vi "挥发酚插入数据.vi"(1 "data":T3 {"单位" items=["ug/L", "mg/L", "ppm", "mg/m3", "cm", "ppb", "ug/m3", "%", "nmol/mol", "umol/mol", "MPN/L", "MPN/100ml", "ng/m3", "NTU", "无量纲", "ms/cm", "us/cm"]}, 2 "挥发酚关键参数":T2, 3 "SN":string, 5 "table":string, 7 "测量模式":T4(ring)=enum."水样测试", 9 "数据类型":string(combo)="N", 11 "error in (no error)":errorcluster) -> (15 "error out":errorcluster)   [LabVIEW 2016, in "挥发酚.lvlib"]
uses:
  <vilib>/Utility/error.llb/DialogType.ctl
panel:
  in  "data2":T1={"时间"=timestamp(0 s since 1904-01-01), "测量模式"="水样测试", "数据类型"="N", "检测值"=0.0, "单位"="mg/L", "数据标识"="N", "X0"=0.0, "标样参考值"=0.0, "跨度值"=0.0, "因子编码"="", "X^2"=0.0, "X"=0.0, "B 2"=0.0, "测量量程"=0.0, "测量检出限"=0.0, "测量精度"=0.0, "测量间隔"=0.0, "消解温度"=0.0, "消解时长"=0.0, "三项式系数"=0.0, "二次多项式系数"=0.0, "曲线斜率"=0.0, "曲线截距"=0.0, "线性相关系数"=0.0, "空白校准时间"=timestamp(0 s since 1904-01-01), "标样校准时间"=timestamp(0 s since 1904-01-01), "测量信号值"=0.0, "稀释倍数"=0.0, "量程系数"=0.0, "LastTime"=timestamp(0 s since 1904-01-01), "量程标识"=""}
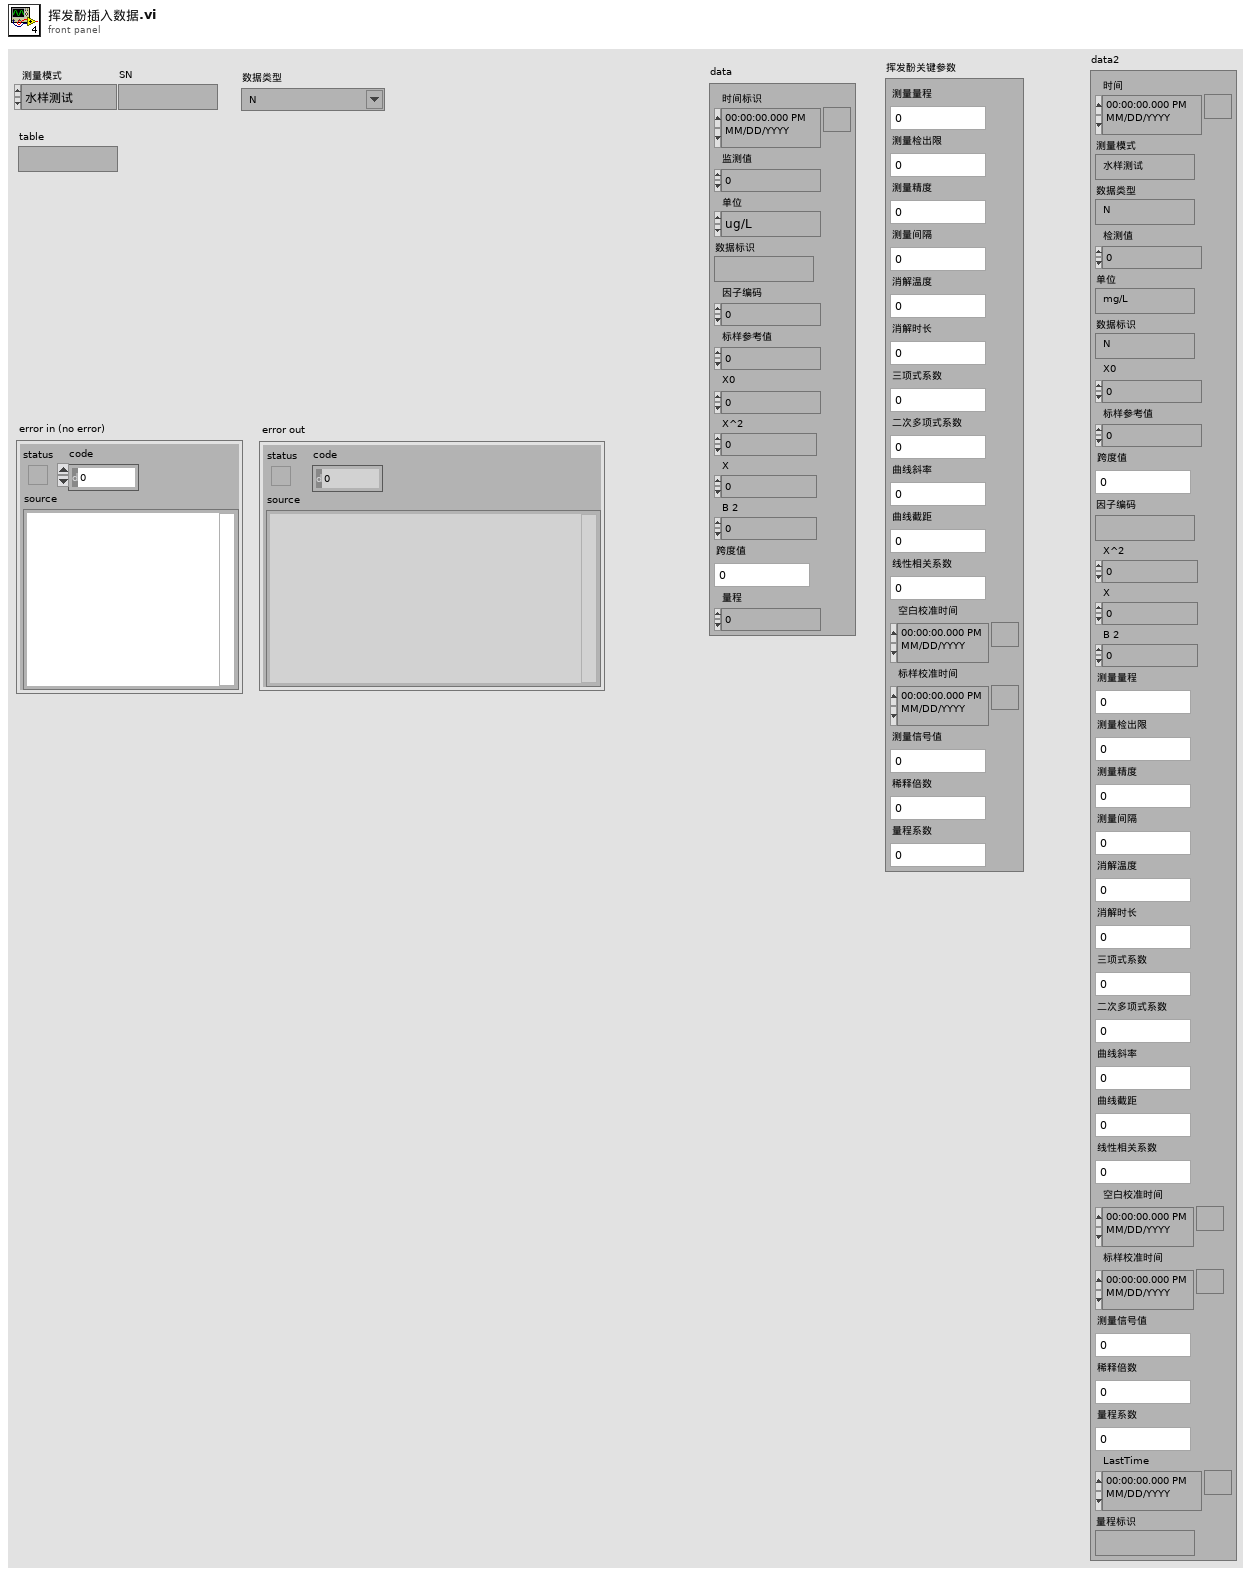
[diagram p1: front panel]
types:
  T1 = cluster{"时间":timestamp, "测量模式":string, "数据类型":string, "检测值":sgl, "单位":string, "数据标识":string, "X0":sgl, "标样参考值":sgl, "跨度值":sgl, "因子编码":string, "X^2":sgl, "X":sgl, "B 2":sgl, "测量量程":sgl, "测量检出限":sgl, "测量精度":sgl, "测量间隔":sgl, "消解温度":sgl, "消解时长":sgl, "三项式系数":sgl, "二次多项式系数":sgl, "曲线斜率":sgl, "曲线截距":sgl, "线性相关系数":sgl, "空白校准时间":timestamp, "标样校准时间":timestamp, "测量信号值":sgl, "稀释倍数":sgl, "量程系数":sgl, "LastTime":timestamp, "量程标识":string}
  T2 = cluster{"测量量程":sgl, "测量检出限":sgl, "测量精度":sgl, "测量间隔":sgl, "消解温度":sgl, "消解时长":sgl, "三项式系数":sgl, "二次多项式系数":sgl, "曲线斜率":sgl, "曲线截距":sgl, "线性相关系数":sgl, "空白校准时间":timestamp, "标样校准时间":timestamp, "测量信号值":sgl, "稀释倍数":sgl, "量程系数":sgl}
  T3 = cluster{"时间标识":timestamp, "监测值":sgl, "单位":u16, "数据标识":string, "因子编码":u32, "标样参考值":sgl, "X0":sgl, "X^2":sgl, "X":sgl, "B 2":sgl, "跨度值":sgl, "量程":sgl}
  T4 = enum16{"维护数据", "水样测试", "标样核查", "零点核查", "跨度核查", "空白测试", "平行样测试", "加标回收", "空白校准", "标样校准", "初始化（清洗）"}
  T5 = typedef "DialogType.ctl" = u16
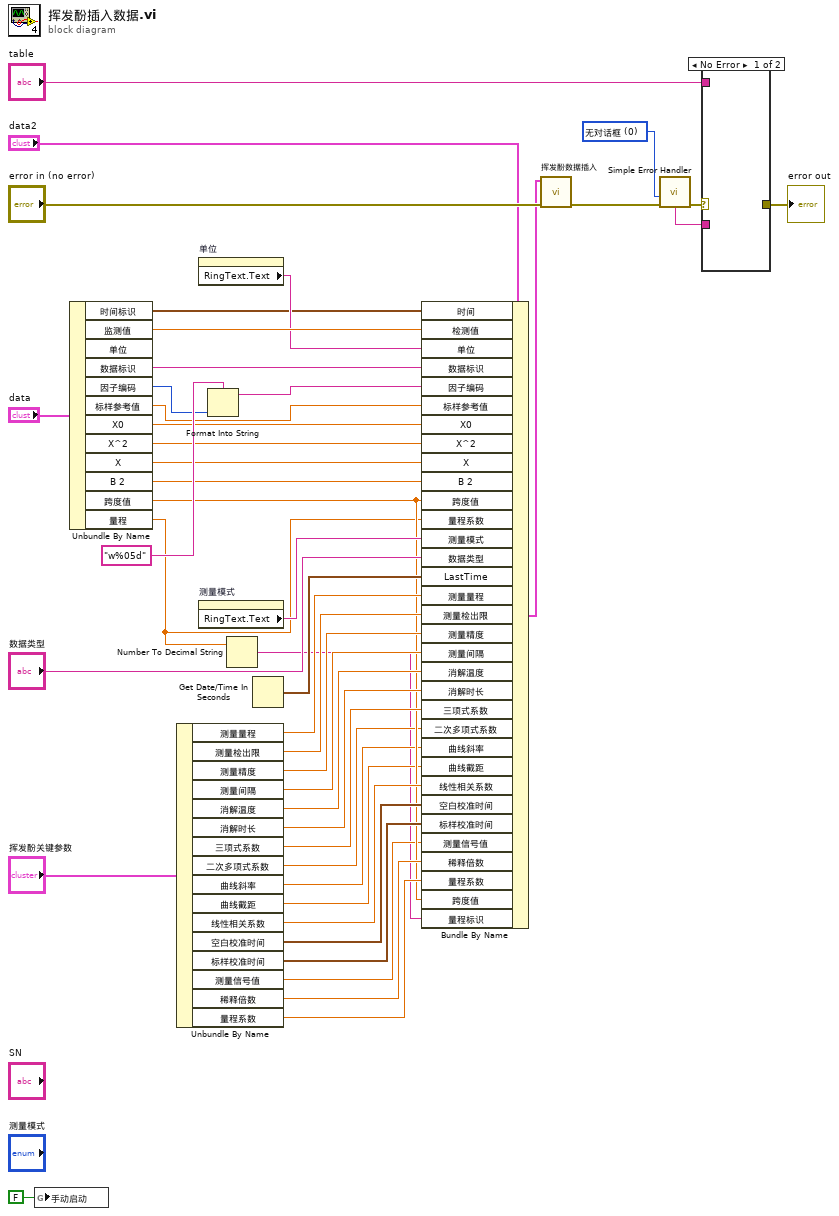
[diagram p0: block diagram]
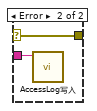
[diagram p2: hidden frame]
diagram:
  w46 = T5 0 items=["无对话框", "确定信息", "继续或停止信息", "确定信息＋警告", "继续/停止+警告"] ("type of dialog (OK msg:1)")
  n1 = global write "VAR挥发酚全局变量.vi" "手动启动"(FALSE ("手动启动")) -> ()
  n2 = Unbundle By Name("data") -> ("时间标识"=w30:timestamp, "监测值"=w40:sgl, "数据标识"=w38:string, "因子编码"=w36:u32, "标样参考值"=w34:sgl, "X0"=w8:sgl, "X^2"=w12:sgl, "X"=w11:sgl, "B 2"=w10:sgl, "跨度值"=w9:sgl, "量程"=w2:sgl)  [unwired: 1 out]
  n3 = Unbundle By Name("挥发酚关键参数") -> ("测量量程"=w29:sgl, "测量检出限"=w28:sgl, "测量精度"=w27:sgl, "测量间隔"=w26:sgl, "消解温度"=w25:sgl, "消解时长"=w24:sgl, "三项式系数"=w23:sgl, "二次多项式系数"=w7:sgl, "曲线斜率"=w6:sgl, "曲线截距"=w5:sgl, "线性相关系数"=w22:sgl, "空白校准时间"=w21:timestamp, "标样校准时间"=w20:timestamp, "测量信号值"=w4:sgl, "稀释倍数"=w19:sgl, "量程系数"=w18:sgl)
  n4 = property on="单位" class="Ring (strict)"() -> ("RingText.Text"=w39:string)  [unwired: 2 in, 2 out]
  n5 = property on="测量模式" class="Enum (strict)"() -> ("RingText.Text"=w33:string)  [unwired: 2 in, 2 out]
  n6 = Format Into String(format string="w%05d" ("格式字符串"), w36) -> (resulting string=w35:string)  [unwired: 2 in, 1 out]
  n7 = Number To Decimal String(number=w2) -> (decimal integer string=w1:string)  [unwired: 1 in]
  n8 = Get Date/Time In Seconds() -> (seconds since 1Jan1904=w31:timestamp)
  n9 = Bundle By Name(cluster="data2", "时间"=w30, "检测值"=w40, "单位"=w39, "数据标识"=w38, "因子编码"=w35, "标样参考值"=w34, "X0"=w8, "X^2"=w12, "X"=w11, "B 2"=w10, "跨度值"=w9, "量程系数"=w2, "测量模式"=w33, "数据类型"="数据类型", "LastTime"=w31, "测量量程"=w29, "测量检出限"=w28, "测量精度"=w27, "测量间隔"=w26, "消解温度"=w25, "消解时长"=w24, "三项式系数"=w23, "二次多项式系数"=w7, "曲线斜率"=w6, "曲线截距"=w5, "线性相关系数"=w22, "空白校准时间"=w21, "标样校准时间"=w20, "测量信号值"=w4, "稀释倍数"=w19, "量程系数"=w18, "跨度值"=w9, "量程标识"=w1) -> (w3:T1)
  n10 = call "挥发酚数据插入.vi"("data"=w3, "错误输入（无错误）"="error in (no error)") -> ("错误输出"=w15:errorcluster)  [unwired: 8 in]
  n11 = call <vilib>:"Simple Error Handler.vi"("type of dialog (OK msg:1)"=w46, "error in (no error)"=w15) -> ("error out"=w45:errorcluster, "message"=w44:string)  [unwired: 3 in, 3 out]
  n12 = case shown="No Error" w45 {
    selector: w45 -> [_ w47]
    tunnel: w44 -> [_ w48]
    tunnel: [_ w47] -> w43
    tunnel: "table" -> [_ _]
    frame No Error {
    }
    frame Error {
      n13 = call "AccessLog写入.vi"("Log"=w48) -> ()  [unwired: 11 in]
    }
  }
  "error out" <- w43
